vi "_Initialize.vi"(8 "error in":errorcluster, 10 "baud rate":u32=57600, 11 "comport":refnum<visa-resource-name>="COM20") -> (0 "error out":errorcluster={"status"=TRUE, "code"=-1073807339, "source"="VISA Read in FirmataClient.lvlib:Initialize.vi"}, 1 "InitializeWasSuccessful":bool, 2 "read":string, 3 "comport out":refnum<visa-resource-name>="COM20", 4 "read data as Array":u8[](array[numeric])=[0, 50, 130, 178, 254] format="%x")   [LabVIEW 2020, in "FirmataClient.lvlib"]
doc: "Initializes comport and makes a request to get the initialization message from the Firmata Protocol."
uses:
  FirmataClient.lvlib
  controls/FirmataProtocolConstants.ctl
  <vilib>/Instr/_visa.llb/VISA Configure Serial Port (Instr).vi
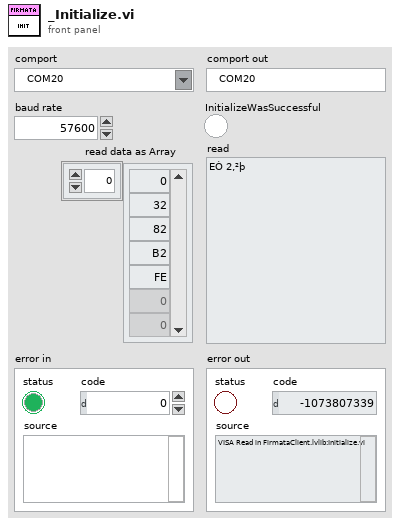
[diagram p1: front panel]
types:
  T1 = typedef "FirmataClient.lvlib/FirmataProtocolConstants.ctl" = u16
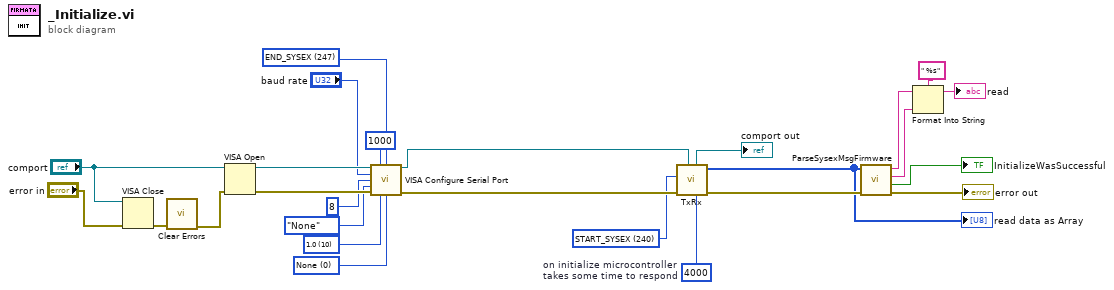
[diagram p0: block diagram]
diagram:
  w4 = T1 240 items=["ANALOG_IO_MESSAGE"=224, "DIGITAL_IO_MESSAGE"=144, "REPORT_ANALOG_PIN"=192, "REPORT_DIGITAL_PORT"=208, "START_SYSEX"=240, "END_SYSEX"=247, "SET_PIN_MODE"=244, "SET_DIGITAL_PIN_VALUE"=245, "PROTOCOL_VERSION"=249, "SYSTEM_RESET"=255, "SYSEX.EXTENDED_ID"=0, "SYSEX.RESERVED_USER_COMMANDs"=1, "SYSEX.ANALOG_MAPPING_QUERY"=105, "SYSEX.ANALOG_MAPPING_RESPONSE"=106, "SYSEX.CAPABILITY_QUERY"=107, "SYSEX.CAPABILITY_RESPONSE"=108, "SYSEX.PIN_STATE_QUERY"=109, "SYSEX.PIN_STATE_RESPONSE"=110, "SYSEX.REPORT_FIRMWARE"=121, "SYSEX.EXTENDED_ANALOG"=111, "SYSEX.STRING_DATA"=113, "SYSEX.REALTIME"=127, "SYSEX.NON_REALTIME"=126, "SYSEX.SAMPLING_INTERVAL"=122] ("FimataProtocolConstants")
  w6 = T1 247 items=["ANALOG_IO_MESSAGE"=224, "DIGITAL_IO_MESSAGE"=144, "REPORT_ANALOG_PIN"=192, "REPORT_DIGITAL_PORT"=208, "START_SYSEX"=240, "END_SYSEX"=247, "SET_PIN_MODE"=244, "SET_DIGITAL_PIN_VALUE"=245, "PROTOCOL_VERSION"=249, "SYSTEM_RESET"=255, "SYSEX.EXTENDED_ID"=0, "SYSEX.RESERVED_USER_COMMANDs"=1, "SYSEX.ANALOG_MAPPING_QUERY"=105, "SYSEX.ANALOG_MAPPING_RESPONSE"=106, "SYSEX.CAPABILITY_QUERY"=107, "SYSEX.CAPABILITY_RESPONSE"=108, "SYSEX.PIN_STATE_QUERY"=109, "SYSEX.PIN_STATE_RESPONSE"=110, "SYSEX.REPORT_FIRMWARE"=121, "SYSEX.EXTENDED_ANALOG"=111, "SYSEX.STRING_DATA"=113, "SYSEX.REALTIME"=127, "SYSEX.NON_REALTIME"=126, "SYSEX.SAMPLING_INTERVAL"=122] ("FimataProtocolConstants")
  w3 = u32 4000  # on initialize microcontroller takes some time to respond
  w19 = u16 0 items=["None", "XON/XOFF", "RTS/CTS", "XON/XOFF & RTS/CTS", "DTR/DSR", "XON/XOFF & DTR/DSR"] ("flow control (0:none)")
  w20 = u16 10 items=["1.0"=10, "1.5"=15, "2.0"=20] ("stop bits (10: 1 bit)")
  n1 = VISA Close(VISA resource name="comport", error in (no error)="error in") -> (error out=w16:errorcluster)
  n2 = call <vilib>:"Clear Errors.vi"("error in (no error)"=w16) -> ("error out"=w15:errorcluster)  [unwired: 5 in, 1 out]
  n3 = VISA Open(error in (no error)=w15, VISA resource name="comport") -> (VISA resource name=w26:refnum<visa-resource-name>, error out=w25:errorcluster)  [unwired: 3 in]
  n4 = call-poly "VISA Configure Serial Port"("VISA resource name"=w26, "timeout (10sec)"=u32 1000, "termination char\n(0xA = '\\n' = LF)"=w6, "baud rate (9600)"="baud rate", "data bits (8)"=u16 8, "parity (0:none)"=enum16{"None", "Odd", "Even", "Mark", "Space"}."None", "error in (no error)"=w25, "stop bits (10: 1 bit)"=w20, "flow control (0:none)"=w19) -> ("VISA resource name out"=w5:refnum<visa-resource-name>, "error out"=w13:errorcluster)  [unwired: 5 in]
  n5 = call "TxRx.vi"("Timeout"=w3, "comport in"=w5, "error in"=w13, "ReplyFirstByte"=w4) -> ("error out"=w12:errorcluster, "ReceivedMessage"=w1:u8[], "comport out"=→"comport out":refnum<visa-resource-name>)  [unwired: 3 in, 2 out]
  "read data as Array" <- w1
  n6 = call "ParseSysexMsgFirmware.vi"("error in"=w12, "Sysex Message"=w1) -> ("error out"=→"error out":errorcluster, "IsValidSysex"=→"InitializeWasSuccessful":bool, "FirmataFirmwareVersion"=w10:string, "FirmataFirmwareName"=w9:string)  [unwired: 6 in]
  n7 = Format Into String(format string=" %s", initial string=w9, w10) -> (resulting string=→"read":string)  [unwired: 1 in, 1 out]
